vi "Set Cell Enabled State.vi"(6 "Disabled State":T1(ring), 8 "error in (no error)":errorcluster, 9 "rowIndex":i32, 10 "colindex":i32, 11 "DataGridView in":refnum<class "DataGridView.lvclass">) -> (0 "error out":errorcluster, 3 "DataGridView out":refnum<class "DataGridView.lvclass">)   [LabVIEW 2014, in "DataGrid.lvlib" / "DataGridView.lvclass"]
doc: "Sets the cell enabled or disabled state. Enabled and Disabled will do simply that, but restore the colors back to the default style and alternating rows default style since the \"Disabled and Grayed\" will grey out the colors and override any customer settings.\n\nCurrently only operates on single cells, 0+ indexing."
uses:
  DataGridView.lvclass
  DataGridView.lvclass/DataGridView.ctl
  System.Windows.Forms
  System.Drawing
  Properties/Read DataGridView.vi
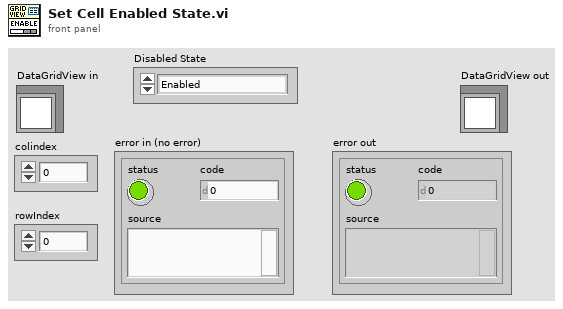
[diagram p1: front panel]
types:
  T1 = enum8{"Enabled", "Disabled", "Disabled and Grayed Out"}
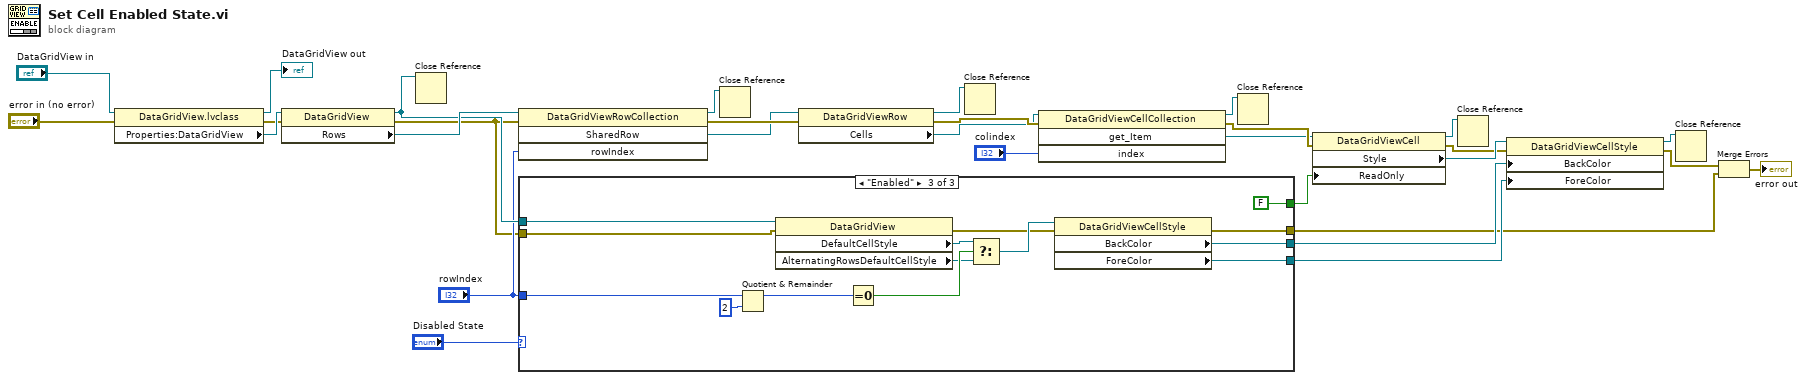
[diagram p0: block diagram]
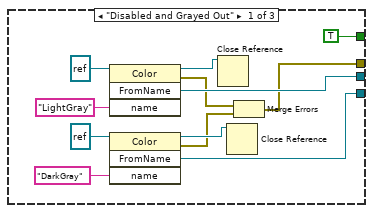
[diagram p2: hidden frame]
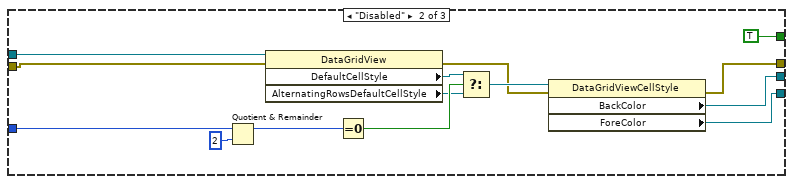
[diagram p3: hidden frame]
diagram:
  n1 = property class="DataGridView.lvclass"(reference="DataGridView in", error in="error in (no error)") -> (reference out=→"DataGridView out":refnum<class "DataGridView.lvclass">, error out=w17:errorcluster, "Properties:DataGridView"=w18:refnum<k24>)
  n2 = property class="DataGridView"(reference=w18, error in=w17) -> (reference out=w7:refnum<k24>, error out=w1:errorcluster, "Rows"=w19:refnum<k24>)
  n3 = Close Reference(reference=w7) -> ()  [unwired: 1 in, 1 out]
  n4 = invoke class="DataGridViewRowCollection" method="SharedRow"(reference=w19, error in=w1, "rowIndex"="rowIndex") -> (reference out=w27:refnum<k24>, error out=w24:errorcluster, "SharedRow"=w20:refnum<k24>)  [unwired: 1 in, 1 out]
  n5 = case shown="\"Enabled\"" "Disabled State" {
    tunnel: [TRUE ("ReadOnly") TRUE ("ReadOnly") FALSE ("ReadOnly")] -> w10
    tunnel: [w37 w54 w68] -> w9
    tunnel: [w36 w53 w67] -> w8
    tunnel: w7 -> [_ w55 w69]
    tunnel: "rowIndex" -> [_ w52 w66]
    tunnel: [w31 w45 w59] -> w2
    tunnel: w1 -> [_ w43 w57]
    frame "Disabled and Grayed Out" {
      n6 = invoke class="Color" method="FromName"(reference=refnum<k24> refnum, "name"="LightGray") -> (reference out=w34:refnum<k24>, error out=w33:errorcluster, "FromName"=w37:refnum<k24>)  [unwired: 2 in, 1 out]
      n7 = invoke class="Color" method="FromName"(reference=refnum<k24> refnum, "name"="DarkGray") -> (reference out=w35:refnum<k24>, error out=w32:errorcluster, "FromName"=w36:refnum<k24>)  [unwired: 2 in, 1 out]
      n8 = Close Reference(reference=w34) -> ()  [unwired: 1 in, 1 out]
      n9 = Close Reference(reference=w35) -> ()  [unwired: 1 in, 1 out]
      n10 = Merge Errors(w33, w32) -> (w31:errorcluster)
    }
    frame "Disabled" {
      n11 = Quotient & Remainder(x=w52, y=2) -> (x-y*floor(x/y)=w50:i32)  [unwired: 1 out]
      n12 = property class="DataGridView"(reference=w55, error in=w43) -> (error out=w44:errorcluster, "DefaultCellStyle"=w48:refnum<k24>, "AlternatingRowsDefaultCellStyle"=w47:refnum<k24>)  [unwired: 1 out]
      n13 = Equal To 0?(x=w50) -> (x = 0?=w49:bool)
      n14 = Select(t=w48, s=w49, f=w47) -> (s? t:f=w46:refnum<k24>)
      n15 = property class="DataGridViewCellStyle"(reference=w46, error in=w44) -> (error out=w45:errorcluster, "BackColor"=w54:refnum<k24>, "ForeColor"=w53:refnum<k24>)  [unwired: 1 out]
    }
    frame "Enabled" {
      n16 = Quotient & Remainder(x=w66, y=2) -> (x-y*floor(x/y)=w64:i32)  [unwired: 1 out]
      n17 = property class="DataGridView"(reference=w69, error in=w57) -> (error out=w58:errorcluster, "DefaultCellStyle"=w62:refnum<k24>, "AlternatingRowsDefaultCellStyle"=w61:refnum<k24>)  [unwired: 1 out]
      n18 = Equal To 0?(x=w64) -> (x = 0?=w63:bool)
      n19 = Select(t=w62, s=w63, f=w61) -> (s? t:f=w60:refnum<k24>)
      n20 = property class="DataGridViewCellStyle"(reference=w60, error in=w58) -> (error out=w59:errorcluster, "BackColor"=w68:refnum<k24>, "ForeColor"=w67:refnum<k24>)  [unwired: 1 out]
    }
  }
  n21 = Close Reference(reference=w27) -> ()  [unwired: 1 in, 1 out]
  n22 = property class="DataGridViewRow"(reference=w20, error in=w24) -> (reference out=w28:refnum<k24>, error out=w25:errorcluster, "Cells"=w21:refnum<k24>)
  n23 = Close Reference(reference=w28) -> ()  [unwired: 1 in, 1 out]
  n24 = invoke class="DataGridViewCellCollection" method="get_Item"(reference=w21, error in=w25, "index"="colindex") -> (reference out=w29:refnum<k24>, error out=w26:errorcluster, "get_Item"=w23:refnum<k24>)  [unwired: 1 in, 1 out]
  n25 = Close Reference(reference=w29) -> ()  [unwired: 1 in, 1 out]
  n26 = property class="DataGridViewCell"(reference=w23, error in=w26, "ReadOnly"=w10) -> (reference out=w30:refnum<k24>, error out=w5:errorcluster, "Style"=w12:refnum<k24>)
  n27 = Close Reference(reference=w30) -> ()  [unwired: 1 in, 1 out]
  n28 = property class="DataGridViewCellStyle"(reference=w12, error in=w5, "BackColor"=w9, "ForeColor"=w8) -> (reference out=w13:refnum<k24>, error out=w4:errorcluster)
  n29 = Close Reference(reference=w13) -> ()  [unwired: 1 in, 1 out]
  n30 = Merge Errors(w4, w2) -> (→"error out":errorcluster)
